vi "Save NI to Configuration File.vi"(5 "NI1":dbl, 7 "NI2":dbl, 11 "error in":errorcluster) -> (15 "error out":errorcluster)   [LabVIEW 2017]
uses:
  <vilib>/Utility/config.llb/Write Key (Double).vi
  <vilib>/Utility/config.llb/NI_LVConfig.lvlib
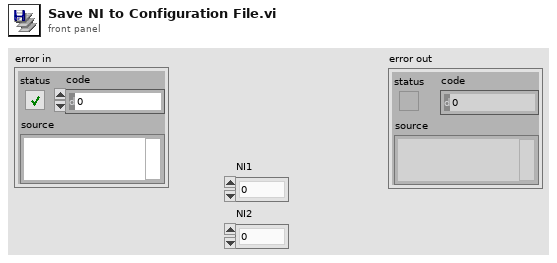
[diagram p1: front panel]
types:
  T1 = typedef "NI_LVConfig.lvlib/Config Data RefNum.ctl" = refnum<k1>
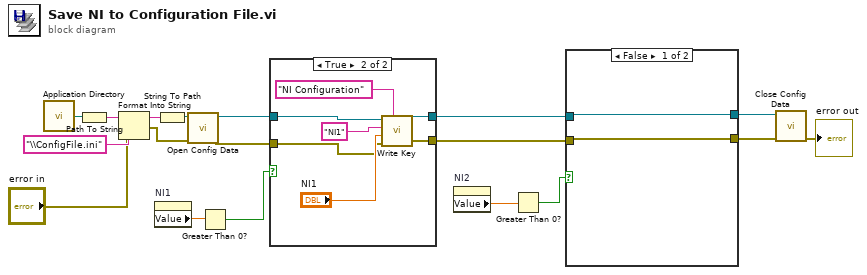
[diagram p0: block diagram]
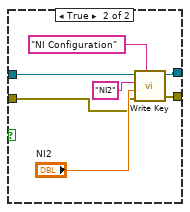
[diagram p2: hidden frame]
diagram:
  n1 = call <vilib>:"Application Directory.vi"() -> ("Application Directory"=w18:path)
  n2 = Path To String(path=w18) -> (string=w17:string)
  n3 = Format Into String(initial string=w17, error in="error in", "\\ConfigFile.ini" ("string")) -> (resulting string=w15:string, error out=w3:errorcluster)  [unwired: 1 in]
  n4 = property on="NI1" class="DigNum (strict)"() -> ("Value"=w7:dbl)  [unwired: 2 in, 2 out]
  n5 = String To Path(string=w15) -> (path=w14:path)
  n6 = call <vilib>:"Open Config Data.vi"("error in (no error)"=w3, "configuration file path"=w14) -> ("error out"=w8:errorcluster, "refnum"=w13:T1)  [unwired: 7 in, 1 out]
  n7 = Greater Than 0?(x=w7) -> (x > 0?=w6:bool)
  n8 = case shown="True" w6 {
    tunnel: w13 -> [w20 w27]
    tunnel: [w20 w24] -> w12
    tunnel: [w19 w22] -> w9
    tunnel: w8 -> [w19 w21]
    frame False {
    }
    frame True {
      n9 = call-poly <vilib>:"Write Key.vi"("section"="NI Configuration", "error in (no error)"=w21, "value"="NI1", "key"="NI1", "refnum"=w27) -> ("error out"=w22:errorcluster, "refnum out"=w24:T1)  [unwired: 4 in, 1 out]
    }
  }
  n10 = property on="NI2" class="DigNum (strict)"() -> ("Value"=w5:dbl)  [unwired: 2 in, 2 out]
  n11 = Greater Than 0?(x=w5) -> (x > 0?=w4:bool)
  n12 = case shown="False" w4 {
    tunnel: w12 -> [w29 w34]
    tunnel: [w29 w32] -> w11
    tunnel: [w28 w31] -> w10
    tunnel: w9 -> [w28 w30]
    frame False {
    }
    frame True {
      n13 = call-poly <vilib>:"Write Key.vi"("section"="NI Configuration", "error in (no error)"=w30, "value"="NI2", "key"="NI2", "refnum"=w34) -> ("error out"=w31:errorcluster, "refnum out"=w32:T1)  [unwired: 4 in, 1 out]
    }
  }
  n14 = call <vilib>:"Close Config Data.vi"("error in (no error)"=w10, "refnum"=w11) -> ("error out"=→"error out":errorcluster)  [unwired: 8 in, 1 out]
